vi "irr-sunrise-equation.vi"(3 "Date":timestamp format="%<%H:%M:%S\n%d/%m/%y>T", 4 "Time Zone (+ to E)":i8 min=-12 max=14, 5 "Longitude (+ to E)":dbl min=-90.0 max=90.0, 6 "Latitude (+ to N)":dbl min=-90.0 max=90.0 format="%#.6f") -> (0 "Solar Elevation Graph":waveform(dbl)(graph), 1 "Sunrise (LST)":timestamp format="%<%H:%M:%S>T", 2 "Sunset (LST)":timestamp format="%<%H:%M:%S>T")   [LabVIEW 2024]
uses:
  <vilib>/express/express arith-compare/Formula/XNode/ExpressFormulaBlockNode.xnode
panel:
  out "points count":i32
  out "Solar Elevation Corr (deg)":dbl
  out "Approx Atm Ref (deg)":dbl
  out "Solar Elevation Angle (deg)":dbl
  out "Solar Zenith Angle (deg)":dbl
  out "Hour Angle (deg)":dbl
  out "True Solar Time (min)":dbl
  out "Time Past Midnight":timestamp format="%<%H:%M:%S\n%d/%m/%y>T"
  out "Sunlight Duration (min)":dbl
  out "Solar Noon (LST)":timestamp format="%<%H:%M:%S>T"
  out "HA Sunrise (deg)":dbl
  out "Eq of Time (min)":dbl
  out "var y":dbl
  out "Sun Declin (deg)":dbl
  out "Sun Rt Ascen (deg)":dbl
  out "Obliq Corr (deg)":dbl
  out "Mean Obliq Ecliptic (deg)":dbl
  out "Sun App Long (deg)":dbl
  out "Sun Rad Vector (AUs)":dbl format="%#.6g"
  out "Sun True Anom (deg)":dbl
  out "Sun True Long (deg)":dbl
  out "Sun Eq of Ctr":dbl format="%#.6g"
  out "Eccent Earth Orbit":dbl format="%#.6g"
  out "Geom Mean Anom Sun (deg)":dbl format="%#.6g"
  out "Geom Mean Long Sun (deg)":dbl format="%#.6g"
  out "Julian Century":dbl format="%#.10g"
  out "Julian Day":dbl format="%#.10g"
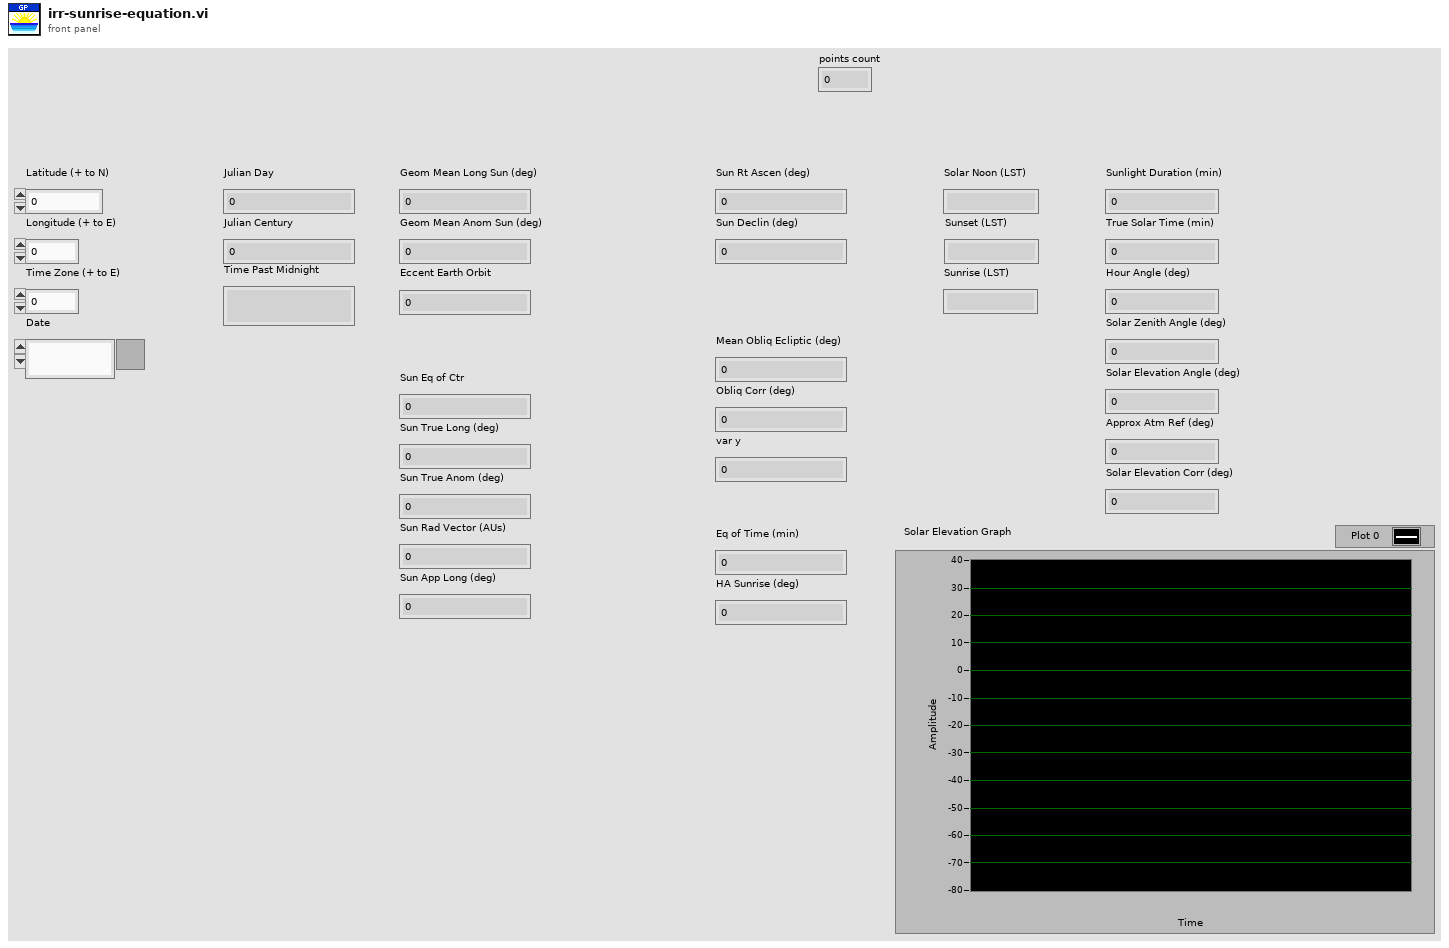
[diagram p1: front panel]
types:
  T1 = typedef "LVDateTimeRec.ctl" = cluster{"fractional second":dbl, "second":i32, "minute":i32, "hour":i32, "day of month":i32, "month":i32, "year":i32, "day of week":i32, "day of year":i32, "DST":i32}
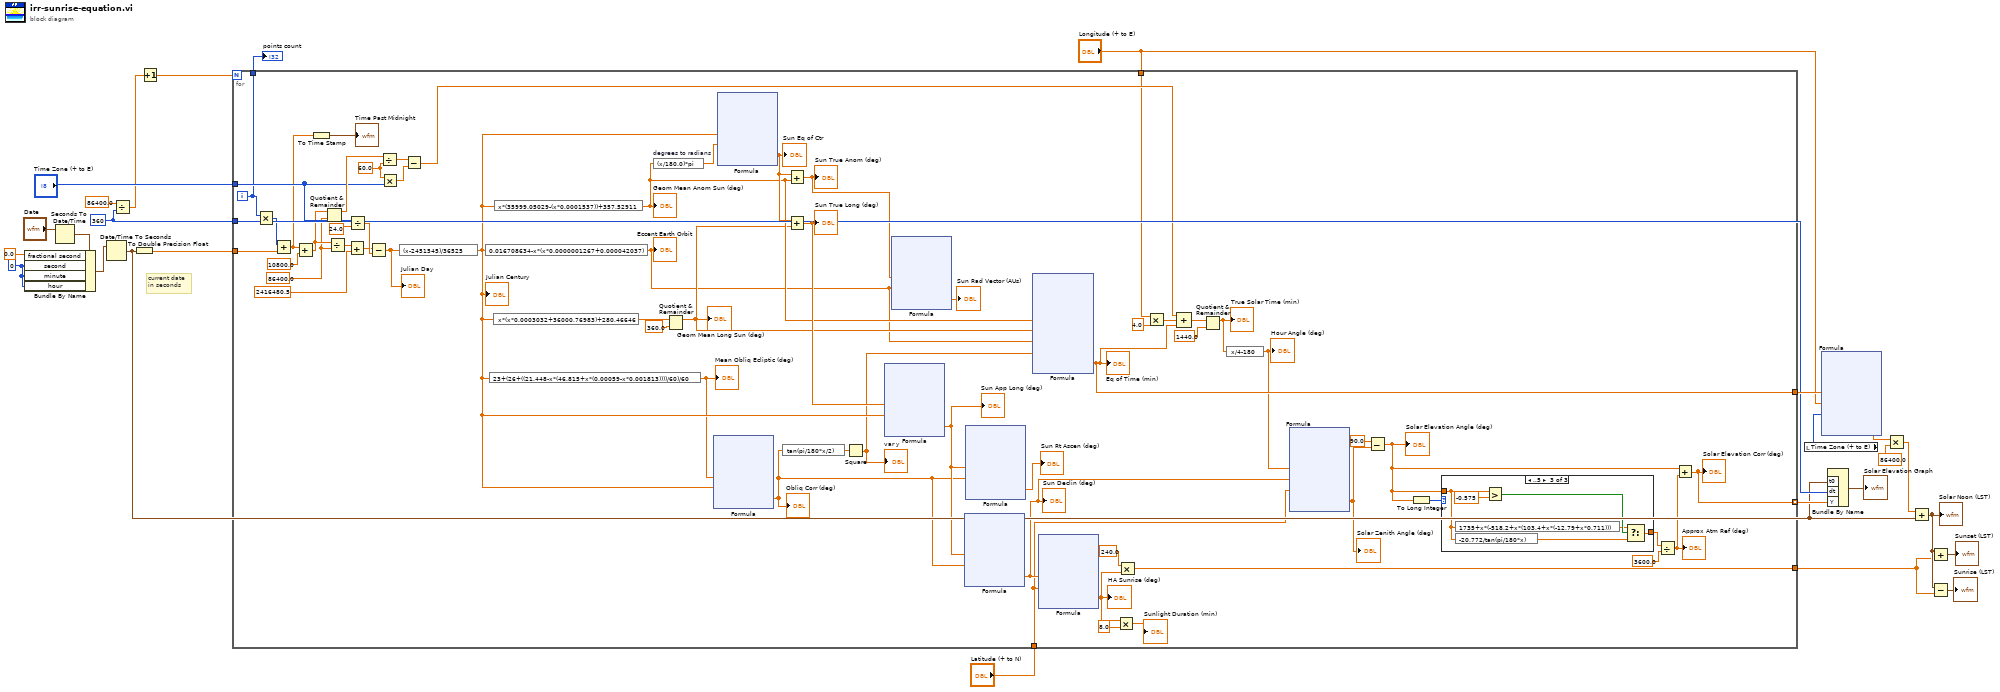
[diagram p0: block diagram]
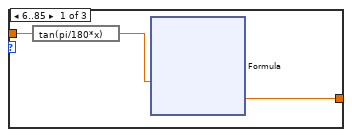
[diagram p2: hidden frame]
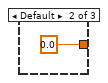
[diagram p3: hidden frame]
diagram:
  w15 = 0 ("second")
  w6 = 360 ("y")
  # "current date \nin seconds"
  n1 = Seconds To Date/Time(time stamp (now)="Date") -> (date time rec=w14:T1)  [unwired: 1 in]
  n2 = Bundle By Name(cluster=w14, "fractional second"=0.0, "second"=w15, "minute"=w15, "hour"=w15) -> (w16:T1)
  n3 = Date/Time To Seconds(2:w16) -> (0:w1:timestamp)  [unwired: 1 in]
  n4 = Divide(x=86400.0 ("y"), y=w6) -> (x/y=w4:dbl)
  n5 = To Double Precision Float(number=w1) -> (double precision float=w12:dbl)
  n6 = Increment(x=w4) -> (x+1=w5:dbl)
  n7 = for {
    N: w5 -> [_]
    tunnel: [w48] -> w26
    tunnel: [w66] -> w20
    tunnel: w6 -> [w64]
    tunnel: w12 -> [w53]
    tunnel: "Time Zone (+ to E)" -> [w37]
    tunnel: "Latitude (+ to N)" -> [w36]
    tunnel: "Longitude (+ to E)" -> [w35]
    tunnel: [w28] -> w8 mode=indexing
    tunnel: [w27] -> w2
    i -> [w27]
    w31 = 86400.0 ("y")
    w51 = 60.0 ("y")
    n8 = Multiply(x=w27, y=w64) -> (x*y=w65:i32)
    n9 = Add(x=w65, y=w53) -> (x+y=w30:dbl)
    n10 = Add(x=w30, y=10800.0) -> (x+y=w33:dbl)
    n11 = To Time Stamp(1:w30) -> (0:→"Time Past Midnight":timestamp)
    n12 = Quotient & Remainder(x=w33, y=w31) -> (x-y*floor(x/y)=w49:dbl)  [unwired: 1 out]
    n13 = Divide(x=w33, y=w31) -> (x/y=w34:dbl)
    n14 = Add(x=w34, y=2416480.5) -> (x+y=w50:dbl)
    n15 = Divide(x=w37, y=24.0) -> (x/y=w86:dbl)
    n16 = Subtract(x=w50, y=w86) -> (x-y=w84:dbl)
    "Julian Day" <- w84
    n17 = Divide(x=w49, y=w51) -> (x/y=w60:dbl)
    n18 = Multiply(x=w51, y=w37) -> (x*y=w59:dbl)
    n19 = expression code="(x-2451545)/36525"(w84) -> (w77:dbl)
    "Julian Century" <- w77
    n20 = Subtract(x=w60, y=w59) -> (x-y=w55:dbl)
    n21 = expression code="0.016708634-x*(x*0.0000001267+0.000042037)"(w77) -> (w68:dbl)
    "Eccent Earth Orbit" <- w68
    n22 = expression code="23+(26+((21.448-x*(46.815+x*(0.00059-x*0.001813))))/60)/60"(w77) -> (w70:dbl)
    "Mean Obliq Ecliptic (deg)" <- w70
    n23 = expression code="x*(x*0.0003032+36000.76983)+280.46646"(w77) -> (w83:dbl)
    n24 = expression code="x*(35999.05029-(x*0.0001537))+357.52911"(w77) -> (w72:dbl)
    "Geom Mean Anom Sun (deg)" <- w72
    n25 = expression code="(x/180.0)*pi" "degrees to radians"(w72) -> (w82:dbl)
    n26 = Quotient & Remainder(x=w83, y=360.0) -> (x-y*floor(x/y)=w71:dbl)  [unwired: 1 out]
    "Geom Mean Long Sun (deg)" <- w71
    n27 = xnode "Formula"("MOE"=w70, "JC"=w77) -> ("Result"=w74:dbl)  [unwired: 1 in, 1 out]
    "Obliq Corr (deg)" <- w74
    n28 = xnode "Formula"("JC"=w77, "GMAS"=w82) -> ("Result"=w81:dbl)  [unwired: 1 in, 1 out]
    "Sun Eq of Ctr" <- w81
    n29 = expression code="tan(pi/180*x/2)"(w74) -> (w73:dbl)
    n30 = Add(x=w81, y=w72) -> (x+y=w78:dbl)
    "Sun True Anom (deg)" <- w78
    n31 = Add(x=w81, y=w71) -> (x+y=w79:dbl)
    "Sun True Long (deg)" <- w79
    n32 = Square(x=w73) -> (x^2=w69:dbl)
    "var y" <- w69
    n33 = xnode "Formula"("STL"=w79, "JC"=w77) -> ("Result"=w75:dbl)  [unwired: 1 in, 1 out]
    "Sun App Long (deg)" <- w75
    n34 = xnode "Formula"("STA"=w78, "EEO"=w68) -> ("Result"=→"Sun Rad Vector (AUs)":dbl)  [unwired: 1 in, 1 out]
    n35 = xnode "Formula"("SAL"=w75, "OC"=w74) -> ("Result"=w45:dbl)  [unwired: 1 in, 1 out]
    "Sun Declin (deg)" <- w45
    n36 = xnode "Formula"("SAL"=w75, "OC"=w74) -> ("Result"=→"Sun Rt Ascen (deg)":dbl)  [unwired: 1 in, 1 out]
    n37 = xnode "Formula"("GMAS"=w72, "GMLS"=w71, "EEO"=w68, "vy"=w69) -> ("Result"=w48:dbl)  [unwired: 1 in, 1 out]
    "Eq of Time (min)" <- w48
    n38 = xnode "Formula"("SD"=w45, "Lat"=w36) -> ("Result"=w63:dbl)  [unwired: 1 in, 1 out]
    "HA Sunrise (deg)" <- w63
    n39 = Multiply(x=w63, y=8.0) -> (x*y=→"Sunlight Duration (min)":dbl)
    n40 = Multiply(x=240.0, y=w63) -> (x*y=w66:dbl)
    n41 = Multiply(x=w35, y=4.0) -> (x*y=w57:dbl)
    n42 = Compound Arithmetic op=ADD(w55, w57, w48) -> (w56:dbl)
    n43 = Quotient & Remainder(x=w56, y=1440.0) -> (x-y*floor(x/y)=w47:dbl)  [unwired: 1 out]
    "True Solar Time (min)" <- w47
    n44 = expression code="x/4-180"(w47) -> (w46:dbl)
    "Hour Angle (deg)" <- w46
    n45 = xnode "Formula"("HA"=w46, "SD"=w45, "Lat"=w36) -> ("Result"=w44:dbl)  [unwired: 1 in, 1 out]
    "Solar Zenith Angle (deg)" <- w44
    n46 = Subtract(x=90.0, y=w44) -> (x-y=w38:dbl)
    "Solar Elevation Angle (deg)" <- w38
    n47 = To Long Integer(number=w38) -> (32bit integer=w42:i32)
    n48 = case shown="..5" w42 {
      tunnel: w38 -> [w90 _ w101]
      tunnel: [w88 0.0 ("x") w100] -> w41
      frame 6..85 {
        n49 = expression code="tan(pi/180*x)"(w90) -> (w89:dbl)
        n50 = xnode "Formula"("TgSEA"=w89) -> ("Result"=w88:dbl)  [unwired: 1 in, 1 out]
      }
      frame Default {
      }
      frame ..5 {
        n51 = expression code="1735+x*(-518.2+x*(103.4+x*(-12.79+x*0.711)))"(w101) -> (w103:dbl)
        n52 = expression code="-20.772/tan(pi/180*x)"(w101) -> (w102:dbl)
        n53 = Greater?(x=w101, y=-0.575) -> (0:w104:bool)
        n54 = Select(t=w103, s=w104, f=w102) -> (s? t:f=w100:dbl)
      }
    }
    n55 = Divide(x=w41, y=3600.0) -> (x/y=w39:dbl)
    "Approx Atm Ref (deg)" <- w39
    n56 = Add(x=w38, y=w39) -> (x+y=w28:dbl)
    "Solar Elevation Corr (deg)" <- w28
  }
  "points count" <- w2
  n57 = local read "Time Zone (+ to E)"() -> (w25:i8)
  n58 = xnode "Formula"("EqT"=w26, "Lon"="Longitude (+ to E)", "TZ"=w25) -> ("Result"=w24:dbl)  [unwired: 1 in, 1 out]
  n59 = Bundle By Name("t0"=w1, "dt"=w6, "Y"=w8) -> (→"Solar Elevation Graph":waveform(dbl))  [unwired: 1 in]
  n60 = Multiply(x=w24, y=86400.0) -> (x*y=w22:dbl)
  n61 = Add(x=w22, y=w1) -> (x+y=w21:timestamp)
  "Solar Noon (LST)" <- w21
  n62 = Add(x=w21, y=w20) -> (x+y=→"Sunset (LST)":timestamp)
  n63 = Subtract(x=w21, y=w20) -> (x-y=→"Sunrise (LST)":timestamp)
